vi "Start Status Reader.vi"(8 "error in (no error)":errorcluster, 11 "Notifier in":refnum<notifier>) -> (0 "error out":errorcluster)   [LabVIEW 2015, in "Tool Module.lvlib"]
uses:
  Tool Module.lvlib
  Tool Interface/_Host - HS Data Stream State Enum Typedef.ctl
  Tool Interface/Tool Interface.lvlib
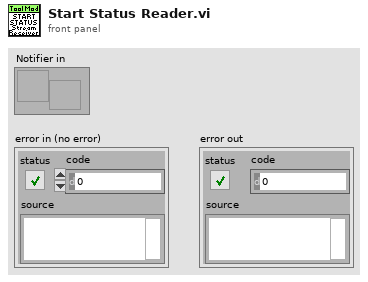
[diagram p1: front panel]
types:
  T1 = typedef "Tool Interface.lvlib/_Host - HS Data Stream State Enum Typedef.ctl" = enum16{"Idle", "Connect", "Receive Data", "Close Connection"}
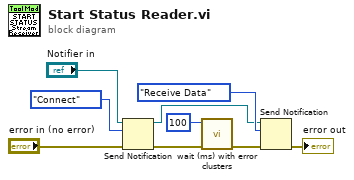
[diagram p0: block diagram]
diagram:
  n1 = Send Notification(notification=_Host_-_HS_Data_Stream_State_Enum_Typedef."Connect", notifier="Notifier in", error in (no error)="error in (no error)") -> (notifier out=w4:refnum<notifier>, error out=w2:errorcluster)
  n2 = call "wait (ms) with error clusters.vi"("error in (no error)"=w2, "milliseconds to wait"=u32 100) -> ("error out"=w1:errorcluster)  [unwired: 9 in]
  n3 = Send Notification(notification=_Host_-_HS_Data_Stream_State_Enum_Typedef."Receive Data", notifier=w4, error in (no error)=w1) -> (error out=→"error out":errorcluster)  [unwired: 1 out]
